vi "cource ns us ns.vi"(3 "ns":i32 min=-1 max=1000, 4 "µs":i32 min=-1 max=1000, 5 "ms":i32) -> (0 "ns out":i32 min=-1 max=1000, 1 "µs out":i32 min=0 max=1000, 2 "ms out":i32)   [LabVIEW 2009, in "CS POLARIS BME DG Client.lvlib"]
uses:
  CS POLARIS BME DG Client.lvlib
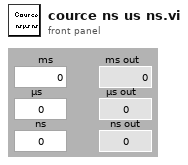
[diagram p1: front panel]
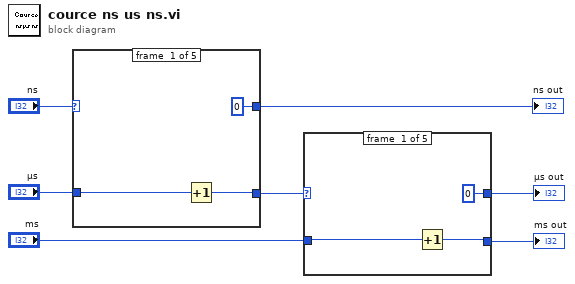
[diagram p0: block diagram]
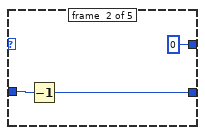
[diagram p2: hidden frame]
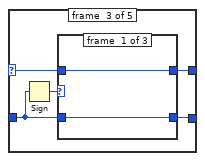
[diagram p3: hidden frame]
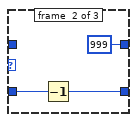
[diagram p4: hidden frame]
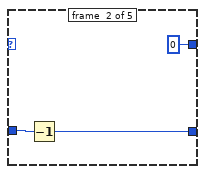
[diagram p8: hidden frame]
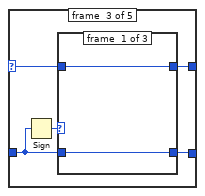
[diagram p9: hidden frame]
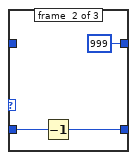
[diagram p10: hidden frame]
diagram:
  n1 = case shown="-999..-1" "ns" {
    selector: "ns" -> [_ _ w15 w27 w29]
    tunnel: [0 ("ns") 0 ("ns") w17 w27 w29] -> w6
    tunnel: "µs" -> [w10 w13 w14 w26 w28]
    tunnel: [w9 w12 w16 w26 w28] -> w3
    frame #0 {
      n2 = Increment(x=w10) -> (x+1=w9:i32)
    }
    frame #1 {
      n3 = Decrement(x=w13) -> (x-1=w12:i32)
    }
    frame #2 {
      n4 = Sign(1:w14) -> (0:w18:i32)
      n5 = case shown="1" w18 {
        tunnel: [w20 999 w25] -> w17
        tunnel: [w19 w22 w24] -> w16
        tunnel: w15 -> [w20 _ w25]
        tunnel: w14 -> [w19 w21 w24]
        frame #0 {
        }
        frame #1 {
          n6 = Decrement(x=w21) -> (x-1=w22:i32)
        }
        frame #2 {
        }
      }
    }
    frame #3 {
    }
    frame #4 {
    }
  }
  "ns out" <- w6
  n7 = case shown="-999..-1" w3 {
    selector: w3 -> [_ _ w37 w49 w51]
    tunnel: [0 ("ns") 0 ("ns") w39 w49 w51] -> w2
    tunnel: "ms" -> [w32 w35 w36 w48 w50]
    tunnel: [w31 w34 w38 w48 w50] -> w1
    frame #0 {
      n8 = Increment(x=w32) -> (x+1=w31:i32)
    }
    frame #1 {
      n9 = Decrement(x=w35) -> (x-1=w34:i32)
    }
    frame #2 {
      n10 = Sign(1:w36) -> (0:w40:i32)
      n11 = case shown="1" w40 {
        tunnel: [w42 999 w47] -> w39
        tunnel: [w41 w44 w46] -> w38
        tunnel: w37 -> [w42 _ w47]
        tunnel: w36 -> [w41 w43 w46]
        frame #0 {
        }
        frame #1 {
          n12 = Decrement(x=w43) -> (x-1=w44:i32)
        }
        frame #2 {
        }
      }
    }
    frame #3 {
    }
    frame #4 {
    }
  }
  "µs out" <- w2
  "ms out" <- w1
